vi "Status Queue.vi"(7 "TcpRouter-Client in":refnum<class "TcpRouter-Client.lvclass">, 8 "error in (no error)":errorcluster) -> (0 "error out":errorcluster, 3 "StatusQueue":refnum<queue>)   [LabVIEW 2020, in "CSM-TCP-Router.lvlib" / "TcpRouter-Client.lvclass"]
uses:
  TcpRouter-Client.lvclass
  Def-TCP-Router Status Data.ctl
  TcpRouter-Client.lvclass/TcpRouter-Client.ctl
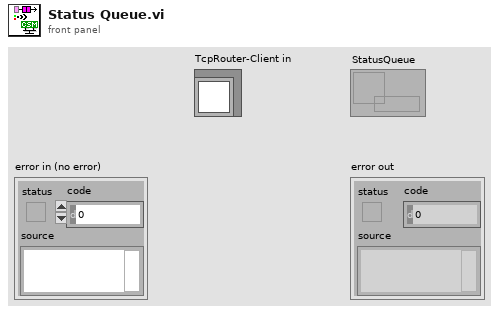
[diagram p1: front panel]
types:
  T1 = cluster{"IP Address":string, "Port":u16, "ConnectTMO":i32}
  T2 = typedef "CSM-TCP-Router.lvlib/TcpRouter-Client.lvclass/Def-TCP-Router Status Data.ctl" = cluster{"status":string, "arg":string, "source":string}
  T3 = typedef "CSM-TCP-Router.lvlib/TcpRouter-Client.lvclass/Def-TCP-Router PUB-SUB.ctl" = cluster{"STATUS":refnum<k5>, "StatusQueue":refnum<queue>}
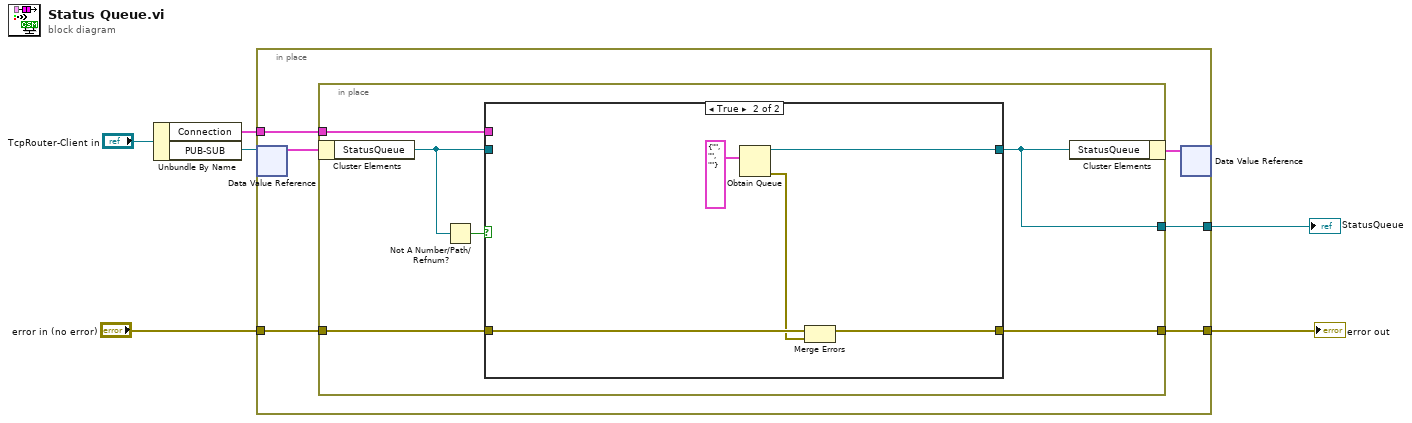
[diagram p0: block diagram]
diagram:
  n1 = Unbundle By Name("TcpRouter-Client in") -> ("Connection"=w2:T1, "PUB-SUB"=w3:refnum<data-value>)
  n2 = in-place {
    in-place-border: w2 -> [w10]
    in-place-border: [w9] -> w5
    in-place-border: "error in (no error)" -> [w8]
    in-place-border: [w7] -> w1
    n3 = in-place-dvr #1(w3) -> (w12:T3)  [unwired: 1 out]
    n4 = in-place {
      in-place-border: w10 -> [w18]
      in-place-border: [w16] -> w9
      in-place-border: w8 -> [w17]
      in-place-border: [w13] -> w7
      n5 = in-place-cluster #2(w12) -> ("StatusQueue"=w14:refnum<queue>)
      n6 = Not A Number/Path/Refnum?(number/path/refnum=w14) -> (NaN/Path/Refnum?=w15:bool)
      n7 = case shown="True" w15 {
        tunnel: w18 -> [_ _]
        tunnel: w17 -> [w19 w25]
        tunnel: [w19 w24] -> w16
        tunnel: [w20 w22] -> w13
        tunnel: w14 -> [w20 _]
        frame False {
        }
        frame True {
          n8 = Obtain Queue(element data type=T2 {"status"="", "arg"="", "source"=""} ("Cluster")) -> (queue out=w22:refnum<queue>, error out=w23:errorcluster)  [unwired: 4 in, 1 out]
          n9 = Merge Errors(w25, w23) -> (w24:errorcluster)
        }
      }
      n10 = in-place-cluster #2("StatusQueue"=w13) -> (w11:T3)
    }
    n11 = in-place-dvr #1(w11) -> ()  [unwired: 2 out]
  }
  "error out" <- w5
  "StatusQueue" <- w1
